vi "Removedoc.vi"() -> ()   [LabVIEW 2021]
panel:
  out "Progress":sgl(slide) scale=0.0..1.0
  out "Name":string
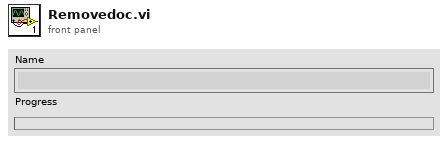
[diagram p1: front panel]
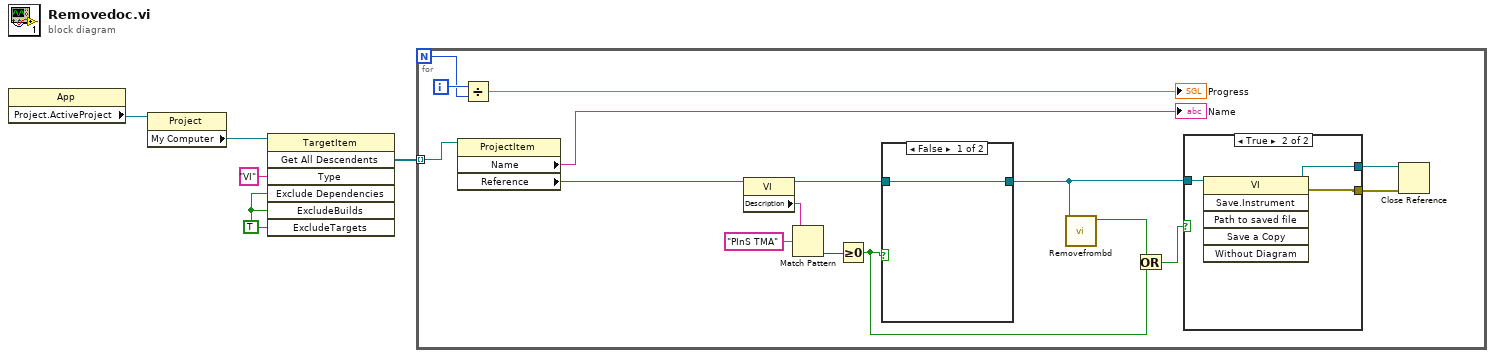
[diagram p0: block diagram]
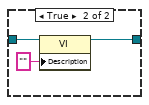
[diagram p3: hidden frame]
diagram:
  w2 = TRUE ("ExcludeTargets")
  n1 = property class="App"() -> ("Project.ActiveProject"=w5:refnum<vi>)  [unwired: 2 in, 2 out]
  n2 = property class="Project"(reference=w5) -> ("My Computer"=w4:refnum<vi>)  [unwired: 1 in, 2 out]
  n3 = invoke class="TargetItem" method="Get All Descendents"(reference=w4, "Type"="VI", "Exclude Dependencies"=w2, "ExcludeBuilds"=w2, "ExcludeTargets"=w2) -> ("All Descendents"=w1:refnum<vi>[])  [unwired: 2 in, 6 out]
  n4 = for {
    N -> [w16]
    tunnel: w1 -> [w20] mode=indexing
    i -> [w17]
    n5 = property class="ProjectItem"(reference=w20) -> ("Name"=→"Name":string, "Reference"=w6:refnum<vi>)  [unwired: 1 in, 2 out]
    n6 = Divide(x=w17, y=w16) -> (x/y=→"Progress":dbl)
    n7 = property class="VI"(reference=w6) -> (reference out=w14:refnum<vi>, "Description"=w13:string)  [unwired: 1 in, 1 out]
    n8 = Match Pattern(string=w13, regular expression="PInS TMA") -> (offset past match=w11:i32)  [unwired: 1 in, 3 out]
    n9 = Greater Or Equal To 0?(x=w11) -> (x >= 0?=w8:bool)
    n10 = case shown="False" w8 {
      tunnel: w14 -> [w26 w29]
      tunnel: [w26 w28] -> w10
      frame False {
      }
      frame True {
        n11 = property class="VI"(reference=w29, "Description"="" ("VI Description")) -> (reference out=w28:refnum<vi>)  [unwired: 1 in, 1 out]
      }
    }
    n12 = call "Removefrombd.vi"("VI Refnum"=w10) -> ("logical OR"=w9:bool)  [unwired: 10 in]
    n13 = Or(x=w9, y=w8) -> (x .or. y?=w7:bool)
    n14 = case shown="True" w7 {
      tunnel: [_ w25] -> w21
      tunnel: [w22 w24] -> w19
      tunnel: w10 -> [w22 w23]
      frame False {
      }
      frame True {
        n15 = invoke class="VI" method="Save.Instrument"(reference=w23) -> (reference out=w24:refnum<vi>, error out=w25:errorcluster)  [unwired: 5 in, 4 out]
      }
    }
    n16 = Close Reference(reference=w19, error in (no error)=w21) -> ()  [unwired: 1 out]
  }
